vi "database_connection_write_DMMS_1.vi"(5 "ODBC data source name":string="amrc_monitoring", 6 "error in (no error)":errorcluster, 7 "G1?":u32, 8 "current time":timestamp, 9 "data 2":dbl[](array[numeric]), 10 "Machine Data":T1={"Zload"="", "Yload"="", "Xload"="", "path_position"="", "Fovr"="", "SspeedOvr"="", "Program Name"="", "Program status"="", "Block of code being executed"="", "Line of code"="", "Machine availability"="", "Emergency status"="", "Controller mode"="", "Tool_id"="UNAVAILABLE"}, 11 "Machine type":string) -> (3 "error out":errorcluster)   [LabVIEW 2017]
uses:
  <vilib>/addons/database/Connection.llb/DB Tools Open Connec (Path).vi
  <vilib>/addons/database/Connection.llb/Conn Execute.vi
  <vilib>/addons/database/Recordset.llb/Rec Destroy - Connection.vi
  <vilib>/addons/database/NI_Database_API.lvlib
panel:
  out "concatenated string 6":string
  out "concatenated string 2":string
  out "resulting string 2":string
  out "ODBC data source name 2":string="amrc_monitoring"
  out "resulting string":string
  out "size(s)":i32
  out "concatenated string 5":string
  out "concatenated string 3":string
  out "concatenated string":string
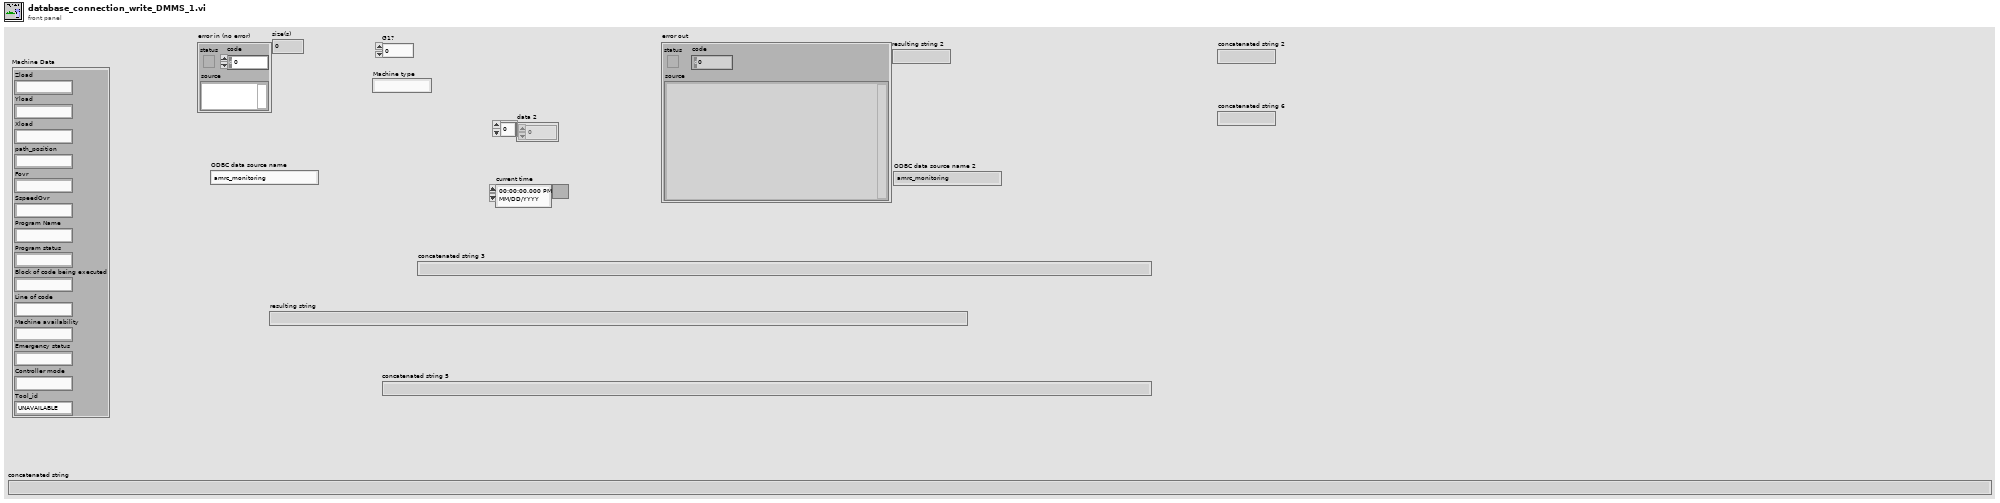
[diagram p1: front panel]
types:
  T1 = cluster{"Zload":string, "Yload":string, "Xload":string, "path_position":string, "Fovr":string, "SspeedOvr":string, "Program Name":string, "Program status":string, "Block of code being executed":string, "Line of code":string, "Machine availability":string, "Emergency status":string, "Controller mode":string, "Tool_id":string}
  T2 = typedef "NI_Database_API.lvlib/Conn ObjectReference.ctl" = refnum<k1>
  T3 = typedef "NI_Database_API.lvlib/Rec ObjectReference.ctl" = refnum<k1>
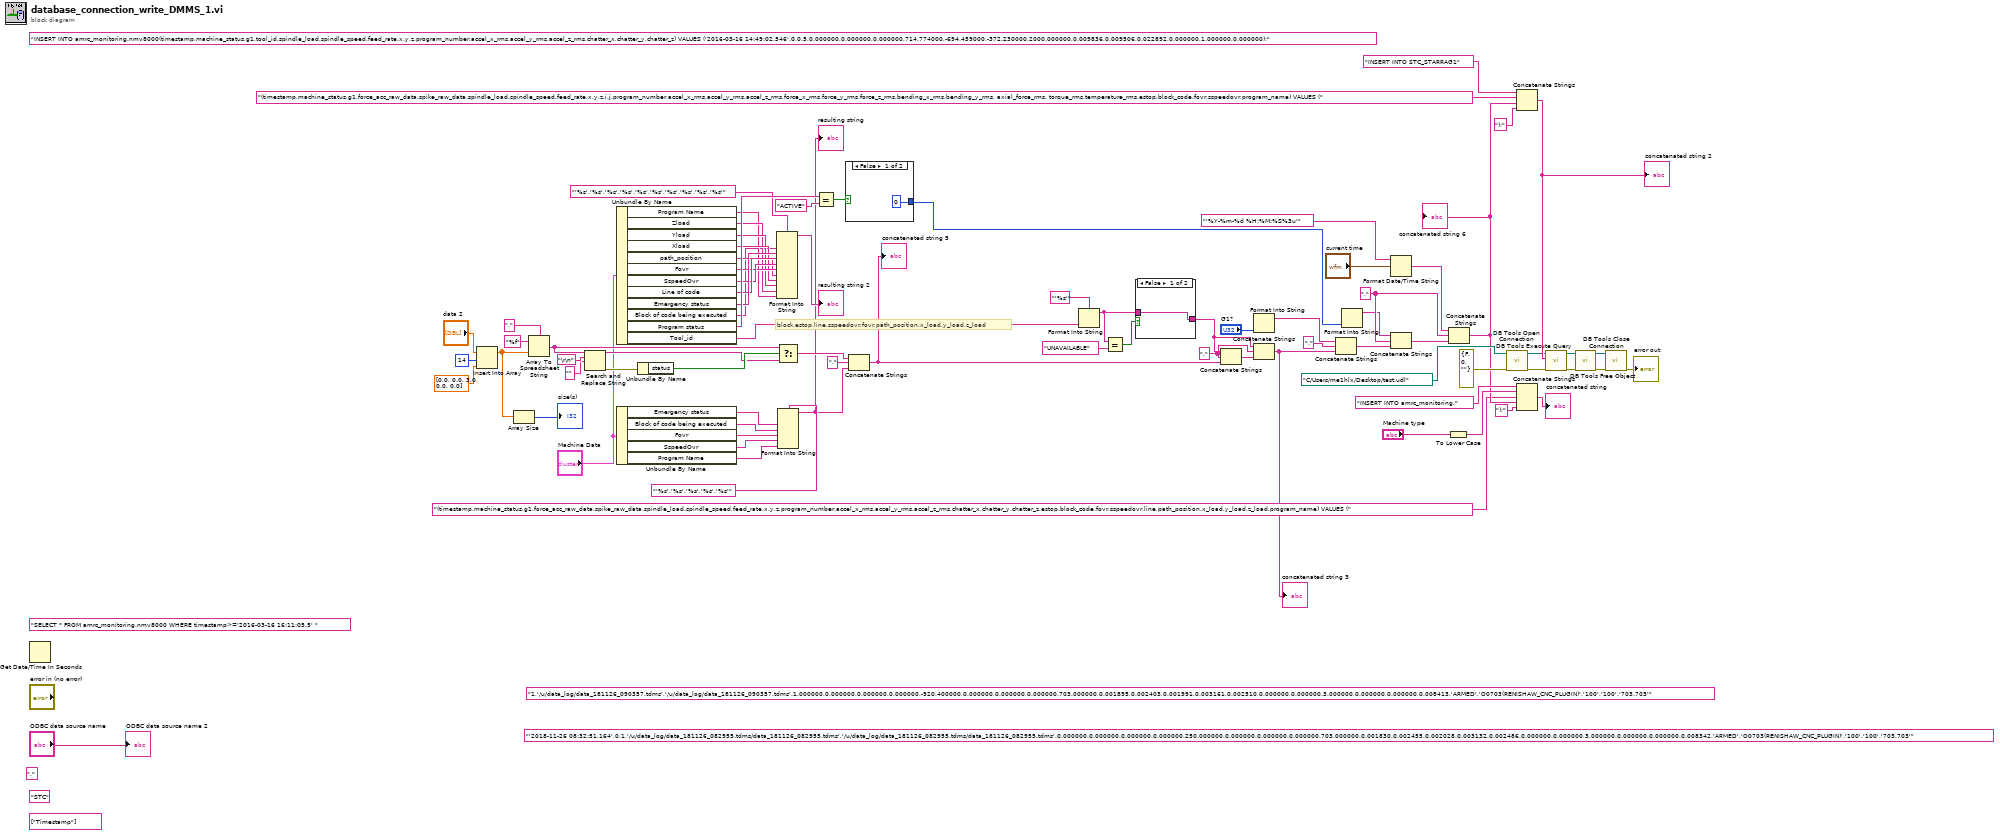
[diagram p0: block diagram]
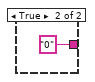
[diagram p2: hidden frame]
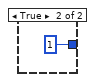
[diagram p3: hidden frame]
diagram:
  (unwired) "1,'/u/data_log/data_181126_090357.tdms','/u/data_log/data_181126_090357.tdms',1.000000,0.000000,0.000000,0.000000,-920.400000,0.000000,0.000000,0.000000,703.000000,0.001895,0.002403,0.001991,0.003161,0.002510,0.000000,0.000000,3.000000,0.000000,0.000000,0.008413,'ARMED','O0703(RENISHAW_CNC_PLUGIN)','100','100','703.703'" ("concatenated string 4")
  (unwired) "'2018-11-26 08:32:51.164',0,1,'/u/data_log/data_181126_082955.tdms/data_181126_082955.tdms','/u/data_log/data_181126_082955.tdms/data_181126_082955.tdms',0.000000,0.000000,0.000000,0.000000,250.000000,0.000000,0.000000,0.000000,703.000000,0.001830,0.002455,0.002028,0.003132,0.002486,0.000000,0.000000,3.000000,0.000000,0.000000,0.008342,'ARMED','O0703(RENISHAW_CNC_PLUGIN)','100','100','703.703'" ("concatenated string 2")
  (unwired) "," ("string")
  (unwired) string[] ["Timestamp"]
  (unwired) "STC"
  w34 = "," ("string")
  w20 = "," ("string")
  (unwired) "SELECT * FROM amrc_monitoring.nmv8000 WHERE timestamp>='2016-03-16 16:11:05.5' " ("SQL query")
  (unwired) "INSERT INTO amrc_monitoring.nmv8000(timestamp,machine_status,g1,tool_id,spindle_load,spindle_speed,feed_rate,x,y,z,program_number,accel_x_rms,accel_y_rms,accel_z_rms,chatter_x,chatter_y,chatter_z) VALUES ('2016-03-16 14:49:02.546',0,0,5,0.000000,0.000000,0.000000,714.774000,-694.459000,-372.230000,2000.000000,0.009836,0.009506,0.022892,0.000000,1.000000,0.000000);" ("SQL query")
  # "block,estop,line,sspeedovr,fovr,path_position,x_load,y_load,z_load"
  n1 = Get Date/Time In Seconds() -> ()  [unwired: 1 out]
  n2 = Insert Into Array(array="data 2", index=14, new element=dbl[] [0.0, 0.0, 3.0, 0.0, 0.0]) -> (w15:dbl[])
  n3 = Array Size(array=w15) -> (size(s)=→"size(s)":i32)
  n4 = Array To Spreadsheet String(delimiter (Tab)=",", array=w15, 3:"%f" ("format string")) -> (spreadsheet string=w64:string)
  n5 = Search and Replace String(input string=w64, search string="\r\n", replace string="" ("replace string (\"\")")) -> (result string=w65:string, error out=w67:errorcluster)  [unwired: 5 in, 2 out]
  n6 = Unbundle By Name("Machine Data") -> ("Program Name"=w48:string, "Zload"=w52:string, "Yload"=w53:string, "Xload"=w54:string, "path_position"=w55:string, "Fovr"=w56:string, "SspeedOvr"=w57:string, "Line of code"=w58:string, "Emergency status"=w59:string, "Block of code being executed"=w46:string, "Program status"=w78:string, "Tool_id"=w39:string)
  n7 = Unbundle By Name("Machine Data") -> ("Emergency status"=w11:string, "Block of code being executed"=w10:string, "Fovr"=w9:string, "SspeedOvr"=w8:string, "Program Name"=w4:string)
  n8 = Unbundle By Name(w67) -> ("status"=w66:bool)
  n9 = Format Into String(format string="'%s','%s','%s','%s','%s','%s','%s','%s','%s','%s'", w46, w59, w58, w57, w56, w55, w54, w53, w52, w48) -> (resulting string=→"resulting string 2":string)  [unwired: 2 in, 1 out]
  n10 = Select(t=w64, s=w66, f=w65) -> (s? t:f=w49:string)
  n11 = Format Into String(format string="'%s','%s','%s','%s','%s'", w11, w10, w9, w8, w4) -> (resulting string=w7:string)  [unwired: 2 in, 1 out]
  "resulting string" <- w7
  n12 = Equal?(x=w78, y="ACTIVE") -> (x = y?=w76:bool)
  n13 = case shown="False" w76 {
    tunnel: [0 1] -> w75
    frame False {
    }
    frame True {
    }
  }
  n14 = Concatenate Strings(w49, "," ("string"), w7) -> (w19:string)
  "concatenated string 5" <- w19
  n15 = Format Into String(format string="'%s'", w39) -> (resulting string=w38:string)  [unwired: 2 in, 1 out]
  n16 = Equal?(x=w38, y="UNAVAILABLE") -> (x = y?=w74:bool)
  n17 = case shown="False" w74 {
    tunnel: w38 -> [w83 _]
    tunnel: [w83 "0"] -> w21
    frame False {
    }
    frame True {
    }
  }
  n18 = Concatenate Strings(w21, w20, w19) -> (w18:string)
  n19 = Format Into String("G1?") -> (resulting string=w32:string)  [unwired: 3 in, 1 out]
  n20 = Concatenate Strings(w21, w20, w18) -> (w44:string)
  "concatenated string 3" <- w44
  n21 = Concatenate Strings(w32, "," ("string"), w44) -> (w1:string)
  n22 = Format Into String(w75) -> (resulting string=w33:string)  [unwired: 3 in, 1 out]
  n23 = Concatenate Strings(w33, w34, w1) -> (w70:string)
  n24 = Format Date/Time String(time format string (%c)="'%Y-%m-%d %H:%M:%S%3u'", seconds (now)="current time") -> (date/time string=w35:string)  [unwired: 1 in]
  n25 = To Lower Case(string="Machine type") -> (all lower case string=w61:string)
  n26 = Concatenate Strings(w35, w34, w70) -> (w5:string)
  "concatenated string 6" <- w5
  n27 = call-poly <vilib>:"DB Tools Open Connection.vi"("error in (no error)"=errorcluster {"status"=FALSE, "code"=0, "source"=""}, "connection information"=path "C:/Users/me1hlx/Desktop/test.udl") -> ("error out"=w30:errorcluster, "connection reference"=w24:T2)  [unwired: 6 in]
  n28 = Concatenate Strings("INSERT INTO STC_STARRAG1" ("string"), "(timestamp,machine_status,g1,force_acc_raw_data,spike_raw_data,spindle_load,spindle_speed,feed_rate,x,y,z,i,j,program_number,accel_x_rms,accel_y_rms,accel_z_rms,force_x_rms,force_y_rms,force_z_rms,bending_x_rms,bending_y_rms, axial_force_rms, torque_rms,temperature_rms,estop,block_code,fovr,sspeedovr,program_name) VALUES (" ("string"), w5, ");" ("string")) -> (w31:string)
  "concatenated string 2" <- w31
  n29 = Concatenate Strings("INSERT INTO amrc_monitoring." ("string"), w61, "(timestamp,machine_status,g1,force_acc_raw_data,spike_raw_data,spindle_load,spindle_speed,feed_rate,x,y,z,program_number,accel_x_rms,accel_y_rms,accel_z_rms,chatter_x,chatter_y,chatter_z,estop,block_code,fovr,sspeedovr,line,path_position,x_load,y_load,z_load,program_name) VALUES (" ("string"), w5, ");" ("string")) -> (→"concatenated string":string)
  n30 = call-poly <vilib>:"DB Tools Execute Query.vi"("error in (no error)"=w30, "SQL query"=w31, "connection reference"=w24) -> ("error out"=w27:errorcluster, "recordset reference"=w28:T3)  [unwired: 5 in]
  n31 = call-poly <vilib>:"DB Tools Free Object.vi"("error in (no error)"=w27, "recordset reference"=w28) -> ("error out"=w25:errorcluster, "connection reference"=w26:T2)  [unwired: 8 in]
  n32 = call <vilib>:"DB Tools Close Connection.vi"("error in (no error)"=w25, "connection reference"=w26) -> ("error out"=→"error out":errorcluster)  [unwired: 5 in]
  "ODBC data source name 2" <- "ODBC data source name"
